vi "avoid lines.vi"(0 "allowed proximity squared":i16) -> ()   [LabVIEW 2010]
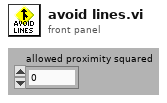
[diagram p1: front panel]
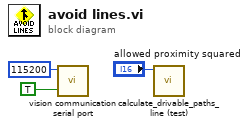
[diagram p0: block diagram]
diagram:
  n1 = call "vision communication serial port.vi"("Invert Polarity?"=TRUE, "baud rate (9600)"=u32 115200) -> ()  [unwired: 10 in]
  n2 = call "calculate_drivable_paths_line (test).vi"("allowed proximity squared"="allowed proximity squared") -> ()  [unwired: 11 in]
